vi "CalibrationAlerts.vi"(9 "Alert Type (0)":i32, 10 "Trigger":bool, 11 "use TLS (True)":bool=TRUE) -> ()   [LabVIEW 2023]
uses:
  Control 1.ctl
  <vilib>/smtpClient/Set Message Text.vi
  <vilib>/smtpClient/LabVIEWSMTPClient.lvlib
panel:
  out "invalid recipients 6":string[](array[string])
  out "invalid recipients 5":string[](array[string])
  out "invalid recipients 4":string[](array[string])
  out "invalid recipients 3":string[](array[string])
  out "invalid recipients 2":string[](array[string])
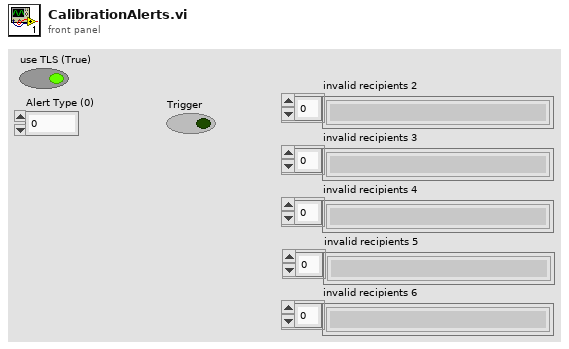
[diagram p1: front panel]
types:
  T1 = typedef "Control 1.ctl" = string
  T2 = typedef "LabVIEWSMTPClient.lvlib/SmtpClientHandle.ctl" = refnum<k1>
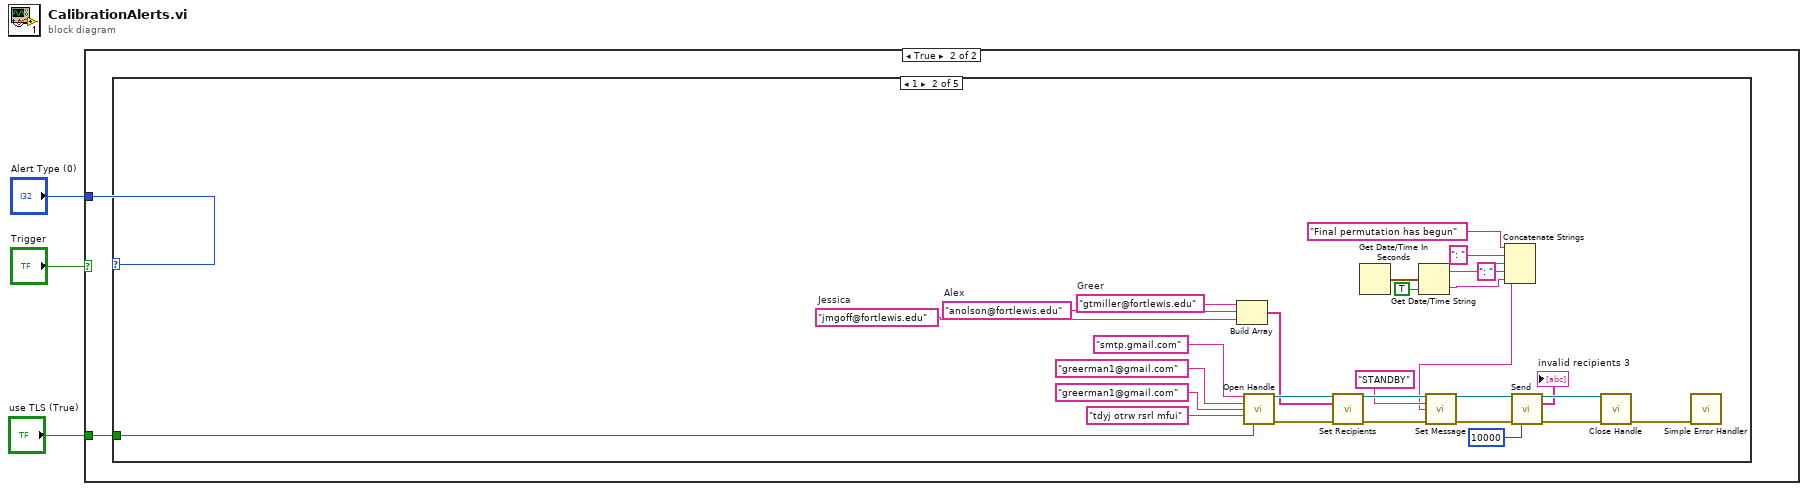
[diagram p0: block diagram]
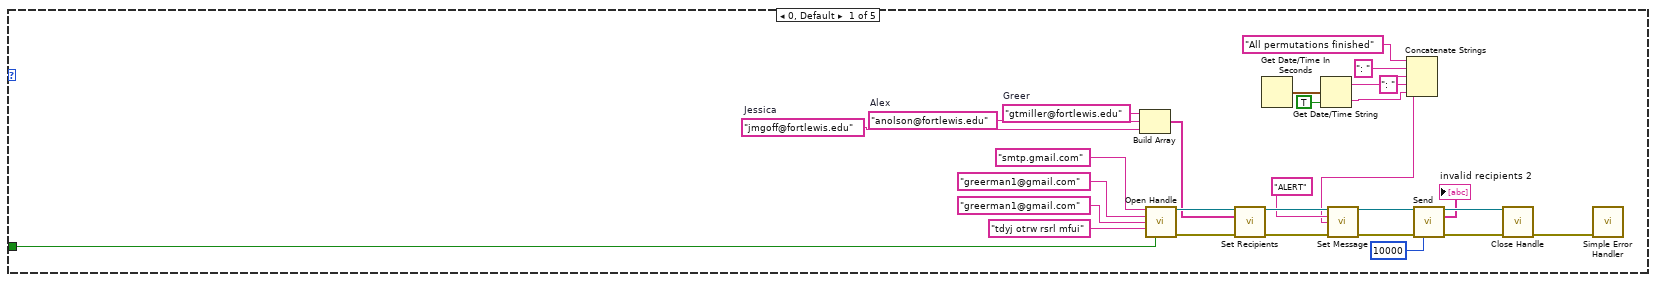
[diagram p3: hidden frame]
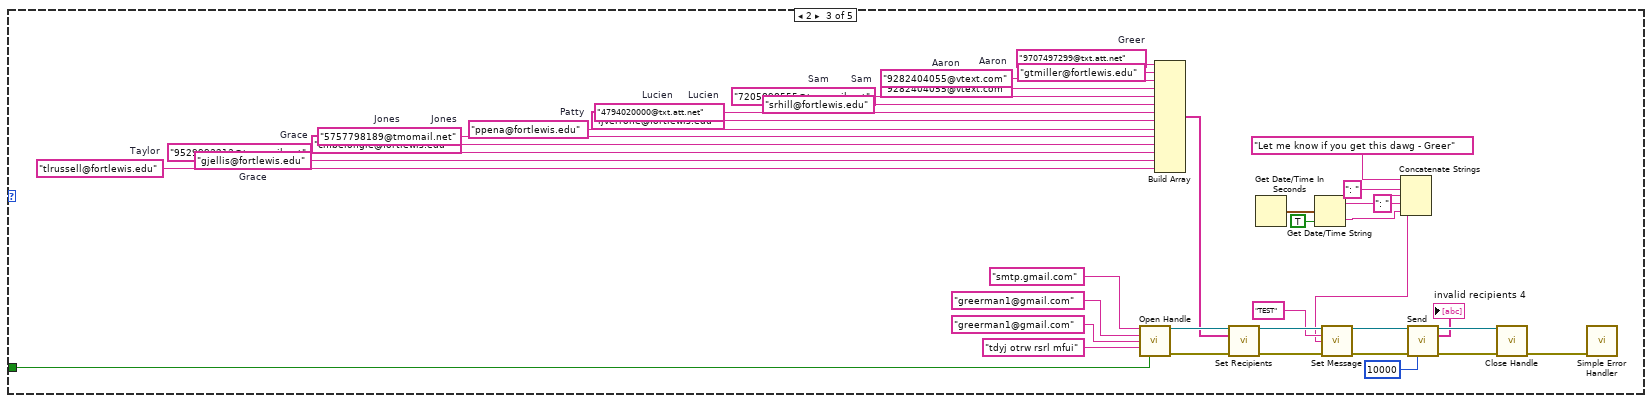
[diagram p4: hidden frame]
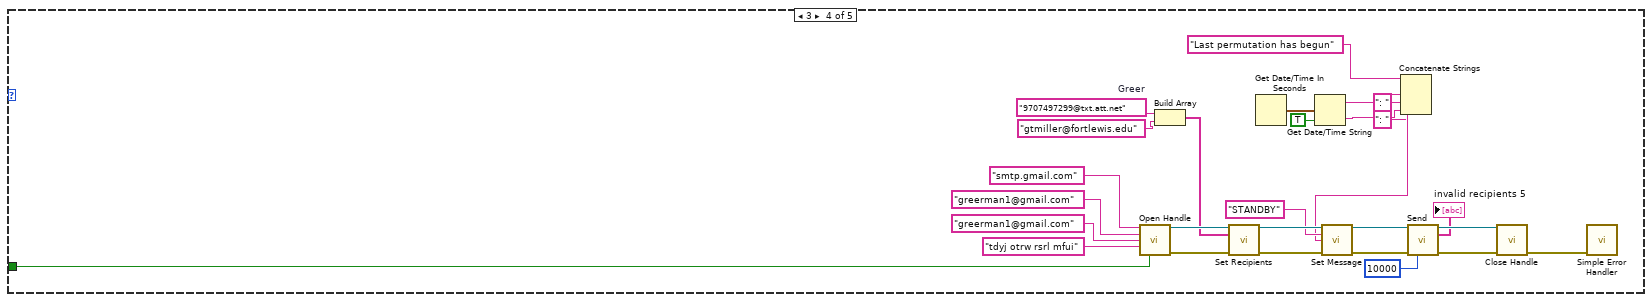
[diagram p5: hidden frame]
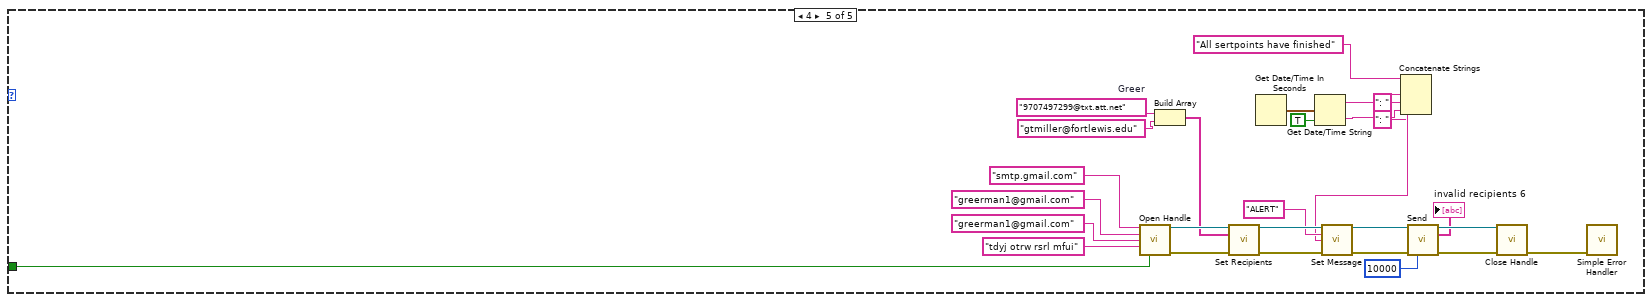
[diagram p6: hidden frame]
diagram:
  n1 = case shown="True" "Trigger" {
    tunnel: "Alert Type (0)" -> [_ w4]
    tunnel: "use TLS (True)" -> [_ w5]
    frame False {
    }
    frame True {
      n2 = case shown="1" w4 {
        tunnel: w5 -> [w18 w41 w80 w108 w136]
        frame 0, Default {
          w6 = "jmgoff@fortlewis.edu"  # Jessica
          w7 = "anolson@fortlewis.edu"  # Alex
          w11 = "gtmiller@fortlewis.edu"  # Greer
          n3 = Build Array(w11, w7, w6) -> (w10:string[])
          n4 = call <vilib>:"Open Handle.vi"("server address"=T1 "smtp.gmail.com" ("server address 2"), "from"="greerman1@gmail.com" ("from 2"), "username"="greerman1@gmail.com" ("username 2"), "password"="tdyj otrw rsrl mfui" ("password 2"), "use TLS (false)"=w18) -> ("handle out"=w27:T2, "error out"=w34:errorcluster)  [unwired: 9 in]
          n5 = call <vilib>:"Set Recipients.vi"("handle in"=w27, "to"=w10, "error in (no error)"=w34) -> ("handle out"=w28:T2, "error out"=w33:errorcluster)  [unwired: 11 in]
          n6 = Get Date/Time In Seconds() -> (seconds since 1Jan1904=w17:timestamp)
          n7 = Get Date/Time String(seconds (now)=w17, want seconds? (F)=TRUE) -> (date string=w14:string, time string=w12:string)  [unwired: 1 in]
          n8 = Concatenate Strings("All permutations finished" ("plain text message 2"), ": " ("string"), w14, ": " ("string"), w12) -> (w15:string)
          n9 = call-poly <vilib>:"Set Message.vi"("handle in"=w28, "subject"="ALERT" ("subject 2"), "plain text message"=w15, "error in (no error)"=w33) -> ("handle out"=w29:T2, "error out"=w32:errorcluster)  [unwired: 10 in]
          n10 = call <vilib>:"Send.vi"("handle in"=w29, "error in (no error)"=w32, "timeout in ms (10000)"=10000) -> ("handle out"=w30:T2, "invalid recipients"=→"invalid recipients 2":string[], "error out"=w31:errorcluster)  [unwired: 10 in]
          n11 = call <vilib>:"Close Handle.vi"("handle in"=w30, "error in (no error)"=w31) -> ("error out"=w26:errorcluster)  [unwired: 12 in, 1 out]
          n12 = call <vilib>:"Simple Error Handler.vi"("error in (no error)"=w26) -> ()  [unwired: 4 in, 5 out]
        }
        frame 1 {
          w35 = "jmgoff@fortlewis.edu"  # Jessica
          w36 = "anolson@fortlewis.edu"  # Alex
          w37 = "gtmiller@fortlewis.edu"  # Greer
          n13 = Build Array(w37, w36, w35) -> (w40:string[])
          n14 = call <vilib>:"Open Handle.vi"("server address"=T1 "smtp.gmail.com" ("server address 2"), "from"="greerman1@gmail.com" ("from 2"), "username"="greerman1@gmail.com" ("username 2"), "password"="tdyj otrw rsrl mfui" ("password 2"), "use TLS (false)"=w41) -> ("handle out"=w56:T2, "error out"=w63:errorcluster)  [unwired: 9 in]
          n15 = call <vilib>:"Set Recipients.vi"("handle in"=w56, "to"=w40, "error in (no error)"=w63) -> ("handle out"=w57:T2, "error out"=w62:errorcluster)  [unwired: 11 in]
          n16 = Get Date/Time In Seconds() -> (seconds since 1Jan1904=w47:timestamp)
          n17 = Get Date/Time String(seconds (now)=w47, want seconds? (F)=TRUE) -> (date string=w44:string, time string=w42:string)  [unwired: 1 in]
          n18 = Concatenate Strings("Final permutation has begun" ("plain text message 2"), ": " ("string"), w44, ": " ("string"), w42) -> (w45:string)
          n19 = call-poly <vilib>:"Set Message.vi"("handle in"=w57, "subject"="STANDBY" ("subject 2"), "plain text message"=w45, "error in (no error)"=w62) -> ("handle out"=w58:T2, "error out"=w61:errorcluster)  [unwired: 10 in]
          n20 = call <vilib>:"Send.vi"("handle in"=w58, "error in (no error)"=w61, "timeout in ms (10000)"=10000) -> ("handle out"=w59:T2, "invalid recipients"=→"invalid recipients 3":string[], "error out"=w60:errorcluster)  [unwired: 10 in]
          n21 = call <vilib>:"Close Handle.vi"("handle in"=w59, "error in (no error)"=w60) -> ("error out"=w55:errorcluster)  [unwired: 12 in, 1 out]
          n22 = call <vilib>:"Simple Error Handler.vi"("error in (no error)"=w55) -> ()  [unwired: 4 in, 5 out]
        }
        frame 2 {
          w68 = "gjellis@fortlewis.edu"  # Grace
          w70 = "cmbelongie@fortlewis.edu"  # Jones
          w73 = "ljverrone@fortlewis.edu"  # Lucien
          w75 = "srhill@fortlewis.edu"  # Sam
          w77 = "9282404055@vtext.com"  # Aaron
          w67 = "tlrussell@fortlewis.edu"  # Taylor
          w69 = "9529993213@tmomail.net"  # Grace
          w71 = "5757798189@tmomail.net"  # Jones
          w72 = "ppena@fortlewis.edu"  # Patty
          w74 = "4794020000@txt.att.net"  # Lucien
          w76 = "7205898555@tmomail.net"  # Sam
          w78 = "9282404055@vtext.com"  # Aaron
          w87 = "9707497299@txt.att.net"  # Greer
          n23 = call <vilib>:"Open Handle.vi"("server address"=T1 "smtp.gmail.com" ("server address 2"), "from"="greerman1@gmail.com" ("from 2"), "username"="greerman1@gmail.com" ("username 2"), "password"="tdyj otrw rsrl mfui" ("password 2"), "use TLS (false)"=w80) -> ("handle out"=w96:T2, "error out"=w103:errorcluster)  [unwired: 9 in]
          n24 = Build Array(w87, "gtmiller@fortlewis.edu", w78, w77, w76, w75, w74, w73, w72, w71, w70, w69, w68, w67) -> (w66:string[])
          n25 = call <vilib>:"Set Recipients.vi"("handle in"=w96, "to"=w66, "error in (no error)"=w103) -> ("handle out"=w97:T2, "error out"=w102:errorcluster)  [unwired: 11 in]
          n26 = Get Date/Time In Seconds() -> (seconds since 1Jan1904=w86:timestamp)
          n27 = Get Date/Time String(seconds (now)=w86, want seconds? (F)=TRUE) -> (date string=w83:string, time string=w81:string)  [unwired: 1 in]
          n28 = Concatenate Strings("Let me know if you get this dawg - Greer" ("plain text message 2"), ": " ("string"), w83, ": " ("string"), w81) -> (w84:string)
          n29 = call-poly <vilib>:"Set Message.vi"("handle in"=w97, "subject"="TEST" ("subject 2"), "plain text message"=w84, "error in (no error)"=w102) -> ("handle out"=w98:T2, "error out"=w101:errorcluster)  [unwired: 10 in]
          n30 = call <vilib>:"Send.vi"("handle in"=w98, "error in (no error)"=w101, "timeout in ms (10000)"=10000) -> ("handle out"=w99:T2, "invalid recipients"=→"invalid recipients 4":string[], "error out"=w100:errorcluster)  [unwired: 10 in]
          n31 = call <vilib>:"Close Handle.vi"("handle in"=w99, "error in (no error)"=w100) -> ("error out"=w95:errorcluster)  [unwired: 12 in, 1 out]
          n32 = call <vilib>:"Simple Error Handler.vi"("error in (no error)"=w95) -> ()  [unwired: 4 in, 5 out]
        }
        frame 3 {
          w115 = "9707497299@txt.att.net"  # Greer
          n33 = call <vilib>:"Open Handle.vi"("server address"=T1 "smtp.gmail.com" ("server address 2"), "from"="greerman1@gmail.com" ("from 2"), "username"="greerman1@gmail.com" ("username 2"), "password"="tdyj otrw rsrl mfui" ("password 2"), "use TLS (false)"=w108) -> ("handle out"=w124:T2, "error out"=w131:errorcluster)  [unwired: 9 in]
          n34 = Build Array(w115, "gtmiller@fortlewis.edu") -> (w106:string[])
          n35 = call <vilib>:"Set Recipients.vi"("handle in"=w124, "to"=w106, "error in (no error)"=w131) -> ("handle out"=w125:T2, "error out"=w130:errorcluster)  [unwired: 11 in]
          n36 = Get Date/Time In Seconds() -> (seconds since 1Jan1904=w114:timestamp)
          n37 = Get Date/Time String(seconds (now)=w114, want seconds? (F)=TRUE) -> (date string=w111:string, time string=w109:string)  [unwired: 1 in]
          n38 = Concatenate Strings("Last permutation has begun" ("plain text message 2"), ": " ("string"), w111, ": " ("string"), w109) -> (w112:string)
          n39 = call-poly <vilib>:"Set Message.vi"("handle in"=w125, "subject"="STANDBY" ("subject 2"), "plain text message"=w112, "error in (no error)"=w130) -> ("handle out"=w126:T2, "error out"=w129:errorcluster)  [unwired: 10 in]
          n40 = call <vilib>:"Send.vi"("handle in"=w126, "error in (no error)"=w129, "timeout in ms (10000)"=10000) -> ("handle out"=w127:T2, "invalid recipients"=→"invalid recipients 5":string[], "error out"=w128:errorcluster)  [unwired: 10 in]
          n41 = call <vilib>:"Close Handle.vi"("handle in"=w127, "error in (no error)"=w128) -> ("error out"=w123:errorcluster)  [unwired: 12 in, 1 out]
          n42 = call <vilib>:"Simple Error Handler.vi"("error in (no error)"=w123) -> ()  [unwired: 4 in, 5 out]
        }
        frame 4 {
          w143 = "9707497299@txt.att.net"  # Greer
          n43 = call <vilib>:"Open Handle.vi"("server address"=T1 "smtp.gmail.com" ("server address 2"), "from"="greerman1@gmail.com" ("from 2"), "username"="greerman1@gmail.com" ("username 2"), "password"="tdyj otrw rsrl mfui" ("password 2"), "use TLS (false)"=w136) -> ("handle out"=w152:T2, "error out"=w159:errorcluster)  [unwired: 9 in]
          n44 = Build Array(w143, "gtmiller@fortlewis.edu") -> (w134:string[])
          n45 = call <vilib>:"Set Recipients.vi"("handle in"=w152, "to"=w134, "error in (no error)"=w159) -> ("handle out"=w153:T2, "error out"=w158:errorcluster)  [unwired: 11 in]
          n46 = Get Date/Time In Seconds() -> (seconds since 1Jan1904=w142:timestamp)
          n47 = Get Date/Time String(seconds (now)=w142, want seconds? (F)=TRUE) -> (date string=w139:string, time string=w137:string)  [unwired: 1 in]
          n48 = Concatenate Strings("All sertpoints have finished" ("plain text message 2"), ": " ("string"), w139, ": " ("string"), w137) -> (w140:string)
          n49 = call-poly <vilib>:"Set Message.vi"("handle in"=w153, "subject"="ALERT" ("subject 2"), "plain text message"=w140, "error in (no error)"=w158) -> ("handle out"=w154:T2, "error out"=w157:errorcluster)  [unwired: 10 in]
          n50 = call <vilib>:"Send.vi"("handle in"=w154, "error in (no error)"=w157, "timeout in ms (10000)"=10000) -> ("handle out"=w155:T2, "invalid recipients"=→"invalid recipients 6":string[], "error out"=w156:errorcluster)  [unwired: 10 in]
          n51 = call <vilib>:"Close Handle.vi"("handle in"=w155, "error in (no error)"=w156) -> ("error out"=w151:errorcluster)  [unwired: 12 in, 1 out]
          n52 = call <vilib>:"Simple Error Handler.vi"("error in (no error)"=w151) -> ()  [unwired: 4 in, 5 out]
        }
      }
    }
  }
